vi "Raycaster_GetSubBufferAddress.vi"(11 "Column":i16) -> (2 "Start Address":i16, 3 "Sub Buffer":u8)   [LabVIEW 2020]
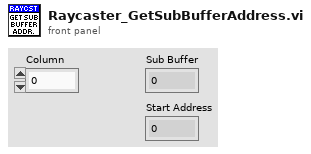
[diagram p1: front panel]
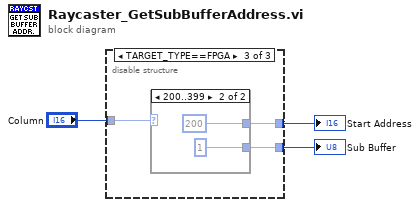
[diagram p0: block diagram]
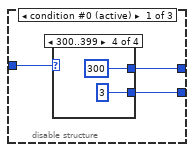
[diagram p2: hidden frame]
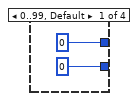
[diagram p3: hidden frame]
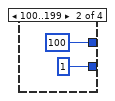
[diagram p4: hidden frame]
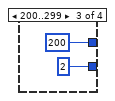
[diagram p5: hidden frame]
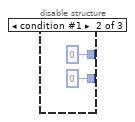
[diagram p6: hidden frame]
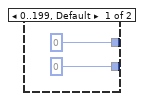
[diagram p7: hidden frame]
diagram:
  n1 = disable-structure shown="TARGET_TYPE==FPGA" {
    disable-tunnel: "Column" -> [w6 _ w19]
    disable-tunnel: [w5 u8 0 ("Sub Buffer") w18] -> w2
    disable-tunnel: [w4 i16 0 ("Start Address") w17] -> w1
    frame condition #0 (active) {
      n2 = case shown="300..399" w6 {
        tunnel: [i16 0 ("y") i16 100 ("y") i16 200 ("y") i16 300 ("y")] -> w4
        tunnel: [u8 0 ("y") u8 1 ("y") u8 2 ("y") u8 3 ("y")] -> w5
        frame 0..99, Default {
        }
        frame 100..199 {
        }
        frame 200..299 {
        }
        frame 300..399 {
        }
      }
    }
    frame condition #1 {
    }
    frame condition #2 {
      n3 = case shown="200..399" w19 {
        tunnel: [i16 0 ("y") i16 200 ("y")] -> w17
        tunnel: [u8 0 ("y") u8 1 ("y")] -> w18
        frame 0..199, Default {
        }
        frame 200..399 {
        }
      }
    }
  }
  "Sub Buffer" <- w2
  "Start Address" <- w1
